vi "Delete.vi"(5 "Delete all found":bool, 6 "$Path or Item Name":string, 7 "error in (no error)":errorcluster, 9 "Offset":i32, 10 "JSON":string="{}") -> (0 "error out":errorcluster, 1 "<JSON> First Deleted Item":string, 2 "Number Deleted":i32, 3 "<JSON>":string caption="<JSON>With Item Deleted")   [LabVIEW 2017, in "JSONtext.lvlib"]
doc: "Deletes JSON item at the JSON Path specified. If \"Delete all found\" is True, will delete all items matching the path. Else will just delete the first found."
uses:
  JSONtext.lvlib
  Parsing/Parsing State.ctl
  support/Quote and Escape JSON string.vi
  Parsing/Advance past whitespace.vi
  support/quote and escape json string 2.vi
  Parsing/Path Notation End Name.vi
  Parsing/Parse Full Path or Item Name.vi
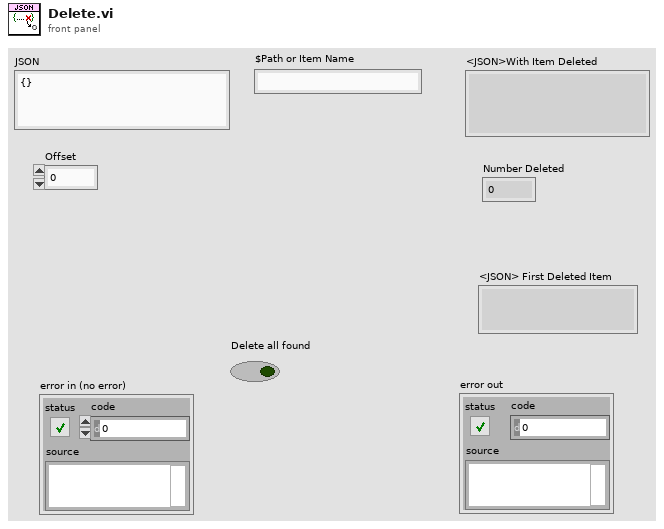
[diagram p1: front panel]
types:
  T1 = typedef "JSONtext.lvlib/Found Items.ctl" = cluster{"Item offset":i32, "Offset past Item":i32, "Name offset":i32, "Offset past Name":i32, "Found":bool, "Item Type":T2, "Item Index":i32}
  T2 = typedef "JSONtext.lvlib/Parsing State.ctl" = enum16{"Parser Error", "Object", "Array", "String", "Number/Other", "Leading Whitespace", "Object end", "Array end", "Value end"}
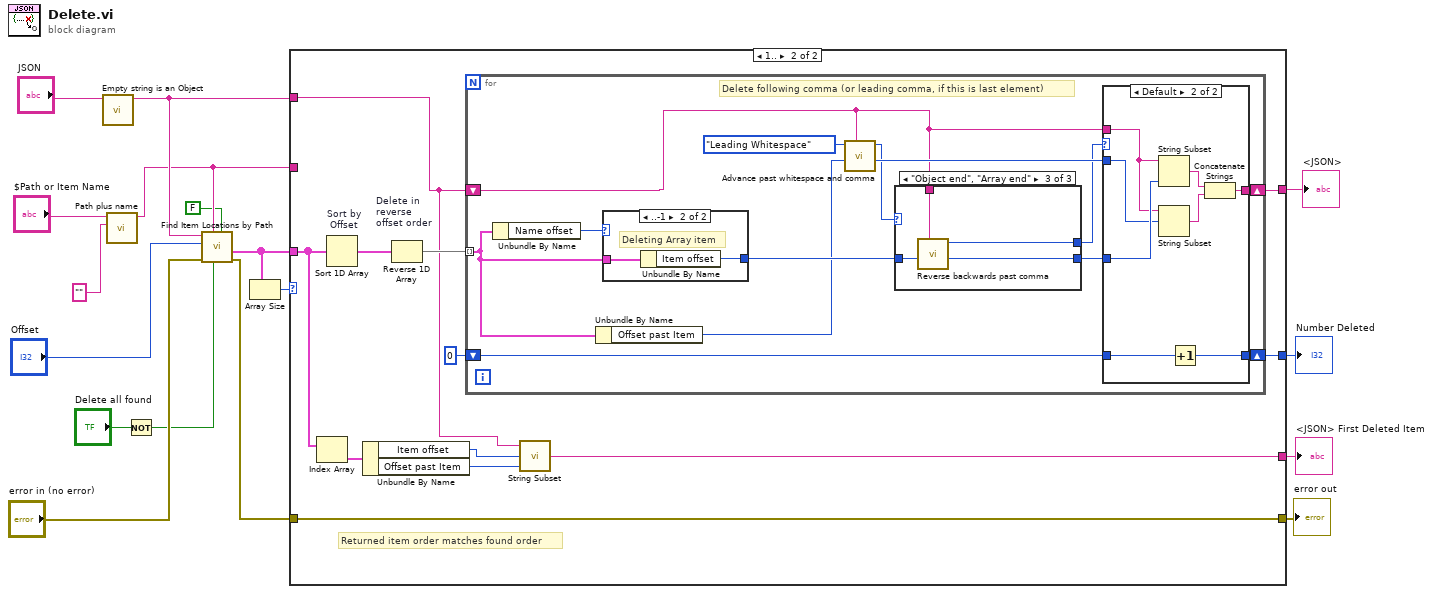
[diagram p0: block diagram]
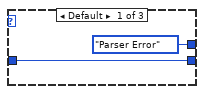
[diagram p5: hidden frame]
diagram:
  n1 = call "Empty string is an Object.vi"("JSON Input"="JSON") -> ("<JSON>Object"=w12:string)  [unwired: 10 in]
  n2 = call "Path plus name.vi"("Item Name"="", "Object (or Item) Path"="$Path or Item Name") -> ("Relative Path or JSON-format name"=w9:string)  [unwired: 6 in, 3 out]
  n3 = Not(x="Delete all found") -> (.not. x?=w2:bool)
  n4 = call "Find Item Locations by Path.vi"("Insertion point if not found"=FALSE, "Only return first found"=w2, "Path"=w9, "error in (no error)"="error in (no error)", "Offset"="Offset", "JSON"=w12) -> ("error out"=w5:errorcluster, "Items"=w7:T1[])  [unwired: 4 in]
  n5 = Array Size(array=w7) -> (size(s)=w6:i32)
  n6 = case shown="1.." w6 {
    tunnel: [w19 w30] -> w17
    tunnel: w12 -> [w19 w21]
    tunnel: w7 -> [_ w23]
    tunnel: w5 -> [w18 w31]
    tunnel: w9 -> [_ _]
    tunnel: [w18 w31] -> w14
    tunnel: [_ w26] -> w3
    tunnel: [_ w20] -> w1
    frame 0, Default {
    }
    frame 1.. {
      # "Returned item order matches found order"
      n7 = Index Array(array=w23) -> (element=w22:T1)  [unwired: 1 in]
      n8 = Sort 1D Array "Sort by\n Offset"(array=w23) -> (sorted array=w28:T1[])
      n9 = Unbundle By Name(w22) -> ("Item offset"=w25:i32, "Offset past Item"=w24:i32)
      n10 = Reverse 1D Array "Delete in \nreverse\noffset order"(array=w28) -> (reversed array=w29:T1[])
      n11 = for {
        tunnel: w29 -> [w36] mode=indexing
        shift-right: [w43] -> w30
        shift-left: w21 -> [w34]
        shift-right: [w33] -> w26
        shift-left: 0 -> [w32]
        # "Delete following comma (or leading comma, if this is last element)"
        n12 = Unbundle By Name(w36) -> ("Name offset"=w38:i32)
        n13 = Unbundle By Name(w36) -> ("Offset past Item"=w35:i32)
        n14 = case shown="..-1" w38 {
          selector: w38 -> [w55 _]
          tunnel: [w55 w57] -> w37
          tunnel: w36 -> [_ w56]
          frame 0.. {
            # "Deleting Object item"
          }
          frame ..-1 {
            # "Deleting Array item"
            n15 = Unbundle By Name(w56) -> ("Item offset"=w57:i32)
          }
        }
        n16 = call "Advance past whitespace and comma.vi"("JSON"=w34, "Offset"=w35, "State in"=Parsing_State."Leading Whitespace") -> ("Offset past match"=w44:i32, "State"=w41:T2)  [unwired: 7 in]
        n17 = case shown="\"Object end\", \"Array end\"" w41 {
          selector: w41 -> [_ w60 _]
          tunnel: w37 -> [w59 w61 w65]
          tunnel: [w59 w61 w64] -> w42
          tunnel: w34 -> [_ _ w63]
          tunnel: [Parsing_State."Parser Error" ("Parser State") w60 w62] -> w40
          frame Default {
          }
          frame "Object".."Number/Other" {
          }
          frame "Object end", "Array end" {
            n18 = call "Reverse backwards past comma.vi"("JSON"=w63, "Offset"=w65) -> ("Offset of first non-whitespace"=w64:i32, "Parser State"=w62:T2)  [unwired: 8 in]
          }
        }
        n19 = case shown="Default" w40 {
          tunnel: w34 -> [w46 w49]
          tunnel: w42 -> [_ w54]
          tunnel: w44 -> [_ w53]
          tunnel: [w46 w50] -> w43
          tunnel: [w45 w48] -> w33
          tunnel: w32 -> [w45 w47]
          frame "Parser Error" {
          }
          frame Default {
            n20 = String Subset(string=w49, length (rest)=w54) -> (substring=w52:string)  [unwired: 1 in]
            n21 = String Subset(string=w49, offset (0)=w53) -> (substring=w51:string)  [unwired: 1 in]
            n22 = Increment(x=w47) -> (x+1=w48:i32)
            n23 = Concatenate Strings(w52, w51) -> (w50:string)
          }
        }
      }
      n24 = call "String Subset.vi"("Offset past End"=w24, "Start offset"=w25, "JSON"=w21) -> ("substring"=w20:string)  [unwired: 2 in]
    }
  }
  "<JSON>" <- w17
  "error out" <- w14
  "Number Deleted" <- w3
  "<JSON> First Deleted Item" <- w1
